vi "Queuevi.vi"() -> ()   [LabVIEW 2015]
panel:
  in  "Stop Button 2":bool
  in  "Numeric 2":dbl
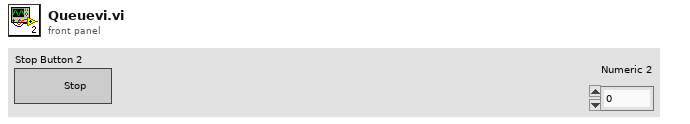
[diagram p1: front panel]
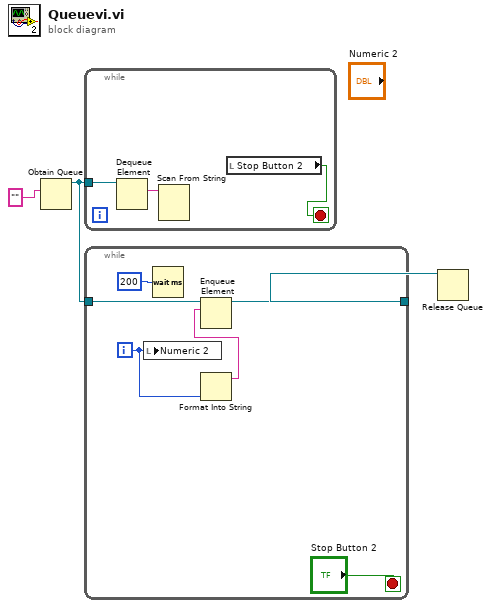
[diagram p0: block diagram]
diagram:
  n1 = Obtain Queue(element data type="") -> (queue out=w3:refnum<queue>)  [unwired: 4 in, 2 out]
  n2 = while {
    tunnel: w3 -> [w6]
    stop <- w4 stop-if-true
    n3 = Dequeue Element(queue=w6) -> (element=w5:string)  [unwired: 2 in, 3 out]
    n4 = Scan From String(input string=w5) -> ()  [unwired: 5 in, 3 out]
    n5 = local read "Stop Button 2"() -> (w4:bool)
  }
  n6 = while {
    tunnel: w3 -> [w11]
    tunnel: [w10] -> w2
    i -> [w9]
    stop <- "Stop Button 2" stop-if-true
    n7 = local write "Numeric 2"(w9) -> ()
    n8 = Wait (ms)(milliseconds to wait=u32 200) -> ()  [unwired: 1 out]
    n9 = Format Into String(w9) -> (resulting string=w8:string)  [unwired: 3 in, 1 out]
    n10 = Enqueue Element(queue=w11, element=w8) -> (queue out=w10:refnum<queue>)  [unwired: 2 in, 2 out]
  }
  n11 = Release Queue(queue=w2) -> ()  [unwired: 2 in, 3 out]
